vi "write_attributes.vi"(8 "error in (no error)":errorcluster caption="entrée d'erreur (pas d'erreur)", 10 "attributes":T1, 11 "Lars en entrée":refnum<class "Lars.lvclass">) -> (0 "error out":errorcluster caption="sortie d'erreur", 3 "Lars en sortie":refnum<class "Lars.lvclass">)   [LabVIEW 2020, in "Lars.lvclass"]
uses:
  Lars.lvclass
  Controls/lars_attributes.ctl
  Lars.lvclass/Lars.ctl
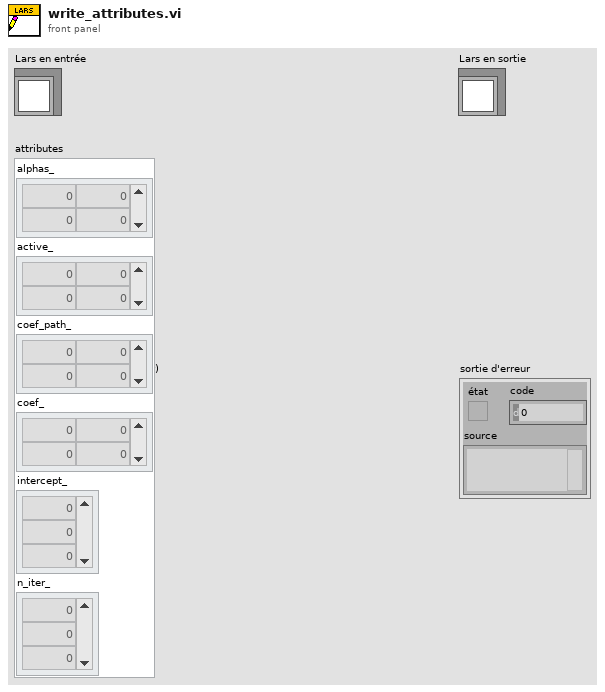
[diagram p1: front panel]
types:
  T1 = typedef "lars_attributes.ctl" = cluster{"alphas_":dbl[][], "active_":dbl[][], "coef_path_":dbl[][][], "coef_":dbl[][], "intercept_":dbl[], "n_iter_":dbl[]}
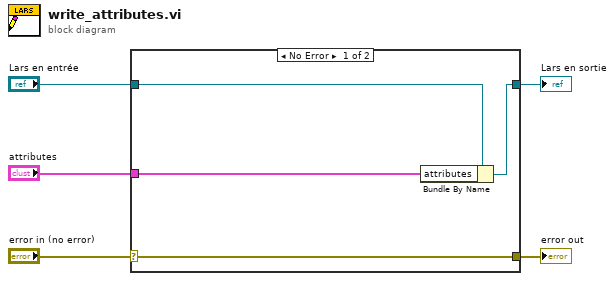
[diagram p0: block diagram]
diagram:
  n1 = case shown="No Error" "error in (no error)" {
    selector: "error in (no error)" -> [w9 w10]
    tunnel: [w9 w10] -> w4
    tunnel: [w7 w11] -> w2
    tunnel: "Lars en entrée" -> [w8 w11]
    tunnel: "attributes" -> [w6 _]
    frame No Error {
      n2 = Bundle By Name(cluster=w8, "attributes"=w6) -> (w7:refnum<class "Lars.lvclass">)
    }
    frame Error {
    }
  }
  "error out" <- w4
  "Lars en sortie" <- w2
